vi "testParseMultipleCommentLines.vi"(8 "error in (no error)":errorcluster, 11 "testStateMachineUtilities in":refnum<class "testStateMachineUtilities.lvclass">) -> (0 "error out":errorcluster, 3 "testStateMachineUtilities out":refnum<class "testStateMachineUtilities.lvclass">)   [LabVIEW 2013, in "testStateMachineUtilities.lvclass"]
uses:
  testStateMachineUtilities.lvclass
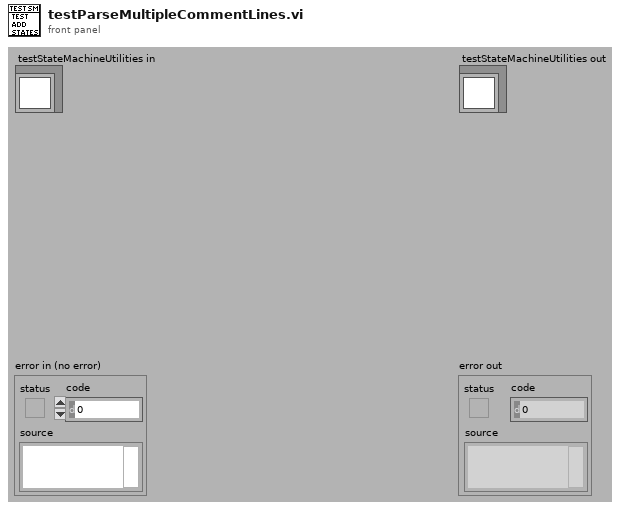
[diagram p1: front panel]
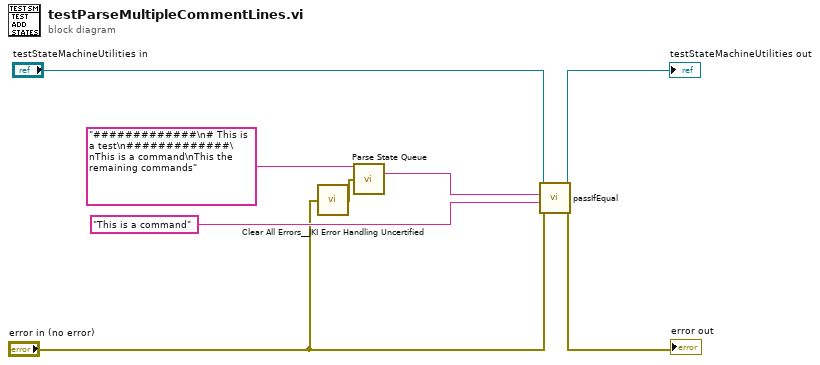
[diagram p0: block diagram]
diagram:
  n1 = call <vilib>:"Clear All Errors__JKI Error Handling Uncertified.vi"("error in"="error in (no error)") -> ("no error out"=w2:errorcluster)  [unwired: 4 in]
  n2 = call "Parse State Queue.vi"("State Queue"="#############\n# This is a test\n#############\nThis is a command\nThis the remaining commands", "Error In (no error)"=w2) -> ("Current State"=w1:string)  [unwired: 11 in, 2 out]
  n3 = call-dynamic "passIfEqual.vi"("error in (no error)"="error in (no error)", "y"="This is a command" ("State Queue"), "x"=w1, "TestCase in"="testStateMachineUtilities in") -> ("error out"=→"error out":errorcluster, "TestCase out"=→"testStateMachineUtilities out":refnum<class "testStateMachineUtilities.lvclass">)  [unwired: 6 in]
